vi "add.publisher.vi"(9 "vol id":i32, 10 "pub id":i32, 11 "pub map in":T1) -> (3 "pub map out":T1)   [LabVIEW 2024, in "manager_daemon.lvclass"]
uses:
  manager_daemon.lvclass
  type_defs/PublisherMap--map.ctl
  type_defs/PublisherData--cluster.ctl
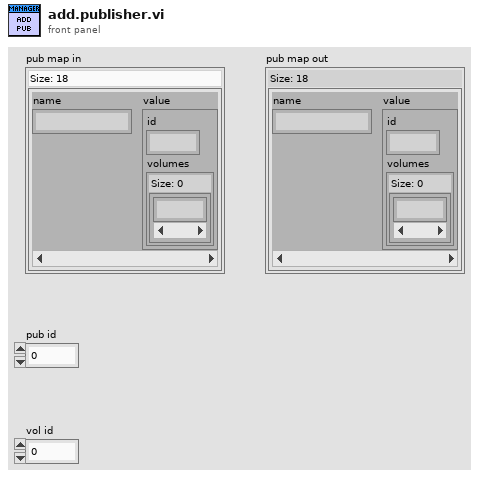
[diagram p1: front panel]
types:
  T1 = typedef "manager_daemon.lvclass/PublisherMap--map.ctl" = map{string, T2}
  T2 = typedef "manager_daemon.lvclass/PublisherData--cluster.ctl" = cluster{"id":i32, "volumes":set{i32}}
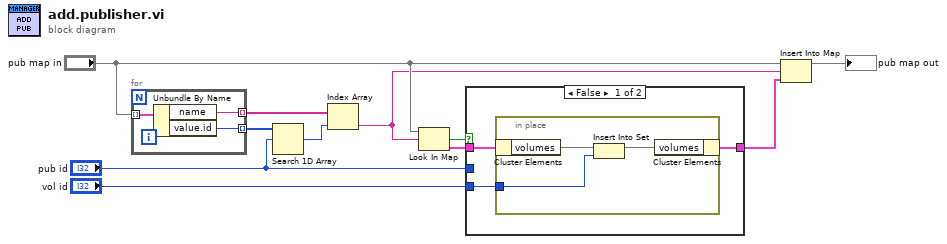
[diagram p0: block diagram]
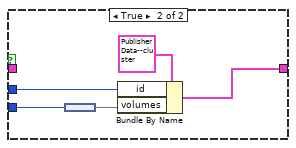
[diagram p2: hidden frame]
diagram:
  n1 = for {
    tunnel: "pub map in" -> [w14] mode=indexing
    tunnel: [w13] -> w5 mode=indexing
    tunnel: [w12] -> w3 mode=indexing
    n2 = Unbundle By Name(w14) -> ("name"=w12:string, "value.id"=w13:i32)
  }
  n3 = Search 1D Array(1D array=w5, element="pub id") -> (index of element=w2:i32)  [unwired: 1 in]
  n4 = Index Array(array=w3, index=w2) -> (element=w1:string)
  n5 = Look In Map(map="pub map in", key=w1) -> (key not found?=w10:bool, value=w9:T2)  [unwired: 1 in]
  n6 = case shown="False" w10 {
    tunnel: w9 -> [w17 _]
    tunnel: "pub id" -> [_ w22]
    tunnel: "vol id" -> [w16 w25]
    tunnel: [w15 w21] -> w7
    frame False {
      n7 = in-place {
        in-place-border: w16 -> [w18]
        n8 = in-place-cluster #1(w17) -> ("volumes"=w20:set{i32})
        n9 = Insert Into Set(10:w18, 11:w20) -> (3:w19:set{i32})  [unwired: 1 out]
        n10 = in-place-cluster #1("volumes"=w19) -> (w15:T2)
      }
    }
    frame True {
      n11 = node(w25) -> (w23:set{i32})
      n12 = Bundle By Name(cluster=T2 {"id"=0, "volumes"={}} ("output cluster"), "id"=w22, "volumes"=w23) -> (w21:T2)
    }
  }
  n13 = Insert Into Map(map in="pub map in", key=w1, value=w7) -> (map out=→"pub map out":T1)  [unwired: 2 out]
